vi "XML ( Set Node Value Multiple Inputs ).vi"(8 "error in (no error)":errorcluster, 9 "Value":string[](array[string]), 10 "XPath expression":string[](array[string]), 11 "XML in":refnum<class "XML.lvclass">) -> (0 "error out":errorcluster, 3 "XML out":refnum<class "XML.lvclass">)   [LabVIEW 2018, in "XML.lvlib" / "XML.lvclass"]
uses:
  XML.lvclass
  XML.lvclass/XML.ctl
  <vilib>/xml/Close Reference(Node).vi
  <vilib>/xml/NI_XML.lvlib
  <resource>/objmgr/DOMUserDefRef.rc
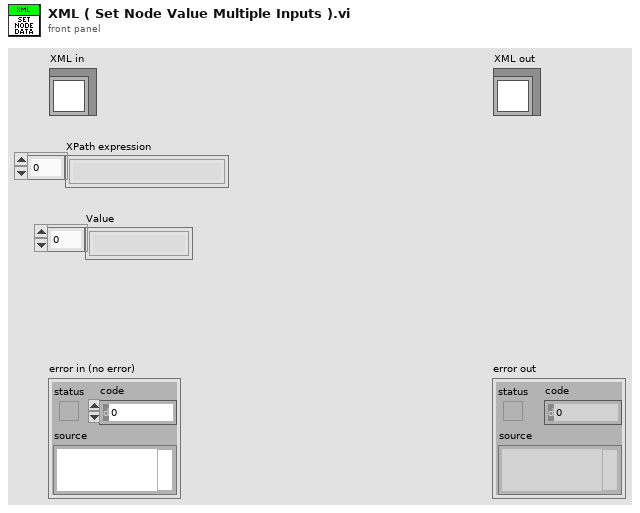
[diagram p1: front panel]
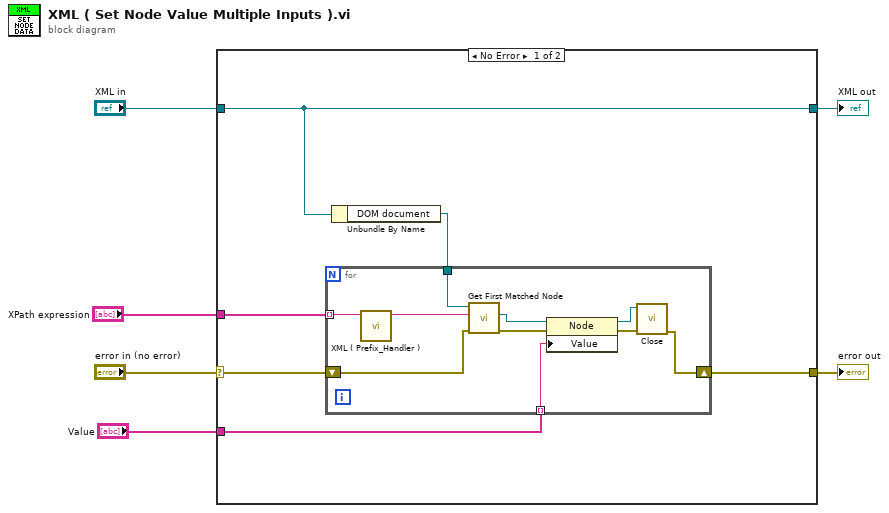
[diagram p0: block diagram]
diagram:
  n1 = case shown="No Error" "error in (no error)" {
    selector: "error in (no error)" -> [w10 w24]
    tunnel: [w9 w24] -> w5
    tunnel: [w12 w23] -> w3
    tunnel: "XML in" -> [w12 w23]
    tunnel: "XPath expression" -> [w8 _]
    tunnel: "Value" -> [w7 _]
    frame No Error {
      n2 = Unbundle By Name(w12) -> ("DOM document"=w11:refnum<k20>)
      n3 = for {
        tunnel: w11 -> [w20]
        tunnel: w8 -> [w15] mode=indexing
        shift-right: [w16] -> w9
        shift-left: w10 -> [w19]
        tunnel: w7 -> [w13] mode=indexing
        n4 = call "XML ( Prefix_Handler ).vi"("input string"=w15) -> ("result string"=w14:string)  [unwired: 10 in]
        n5 = call <vilib>:"Get First Matched Node.vi"("error in (no error)"=w19, "XPath expression"=w14, "node in"=w20) -> ("error out"=w21:errorcluster, "node result"=w22:refnum<k20>)  [unwired: 6 in, 1 out]
        n6 = property class="Node"(reference=w22, error in=w21, "Value"=w13) -> (reference out=w17:refnum<k20>, error out=w18:errorcluster)
        n7 = call-poly <vilib>:"Close.vi"("error in (no error)"=w18, "node"=w17) -> ("error out"=w16:errorcluster)  [unwired: 7 in]
      }
    }
    frame Error {
    }
  }
  "error out" <- w5
  "XML out" <- w3
